vi "Stop Core.vi"(10 "final error code":i32, 11 "Hardware_panel in":refnum<class "thorlabs_panel.lvclass">) -> (3 "Hardware_panel out":refnum<class "thorlabs_panel.lvclass">)   [LabVIEW 2015, in "thorlabs_panel.lvclass"]
doc: "(<B>Filename</B>: Actor Framework.lvlib:Actor.lvclass:Stop Core.vi)\n\nDefines what the actor does before it stops. Use the <B>final error code</B> input to determine whether the actor shut down in response to an error.\n\nBy default, this method does nothing. A descendant class may override it to define behavior, such as shutting down any processes the actor initiated in its override of the Actor Core method."
uses:
  thorlabs_panel.lvclass
  UI/panel_class/panel.lvclass/panel.ctl
  UI/panel_class/panel.lvclass
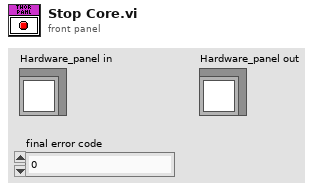
[diagram p1: front panel]
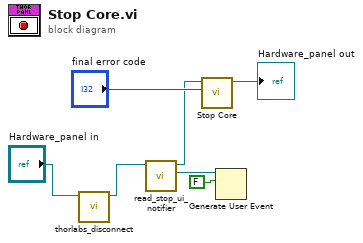
[diagram p0: block diagram]
diagram:
  n1 = call "thorlabs_disconnect.vi"("thorlabs_panel in"="Hardware_panel in") -> ("thorlabs_panel out"=w1:refnum<class "thorlabs_panel.lvclass">)  [unwired: 9 in, 1 out]
  n2 = call "read_stop_ui_notifier.vi"("panel in"=w1) -> ("stop_ui_notifier"=w5:refnum<user-event>, "panel out"=w3:refnum<class "thorlabs_panel.lvclass">)  [unwired: 8 in, 1 out]
  n3 = call-parent "Stop Core.vi"("final error code"="final error code", "Actor in"=w3) -> ("Actor out"=→"Hardware_panel out":refnum<class "thorlabs_panel.lvclass">)  [unwired: 9 in]
  n4 = Generate User Event(user event=w5, event data cluster=FALSE ("event data")) -> ()  [unwired: 2 in, 2 out]
